vi "FEA_Model_Bounded_Regression.vi"(8 "error in (no error)":errorcluster, 11 "FEA_Model in":refnum<class "FEA_Model.lvclass">) -> (0 "error out":errorcluster, 3 "FEA_Model out":refnum<class "FEA_Model.lvclass">)   [LabVIEW 2021, in "FEA_Model.lvclass"]
uses:
  FEA_Model.lvclass
  FEA_Model.lvclass/FEA_Model.ctl
  <vilib>/Analysis/baseanly.llb/Real A x B.vi
  <vilib>/Analysis/baseanly.llb/Real Inverse Matrix.vi
  <vilib>/Analysis/NI_AALBase.lvlib
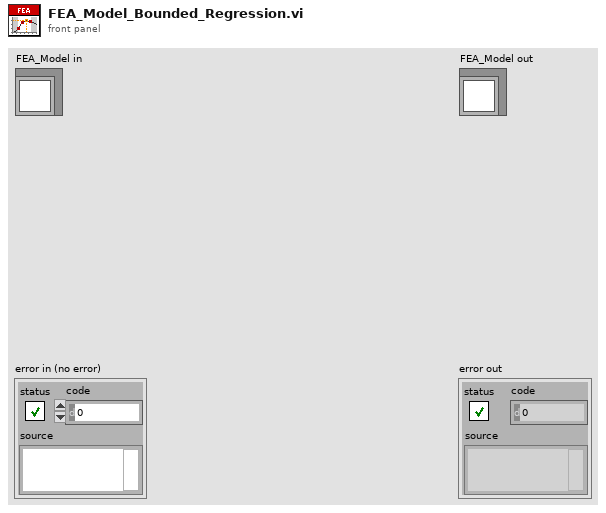
[diagram p1: front panel]
types:
  T1 = enum16{"Scalar Particle to Meter", "Scalar Node to Meter", "Scalar Meter to Particle", "Scalar Meter to Node", "Array Particle to Meter", "Array Node to Meter", "Array Meter to Particle", "Array Meter to Node"}
  T2 = typedef "NI_Matrix.lvlib/RealMatrix.ctl" = dbl[][]
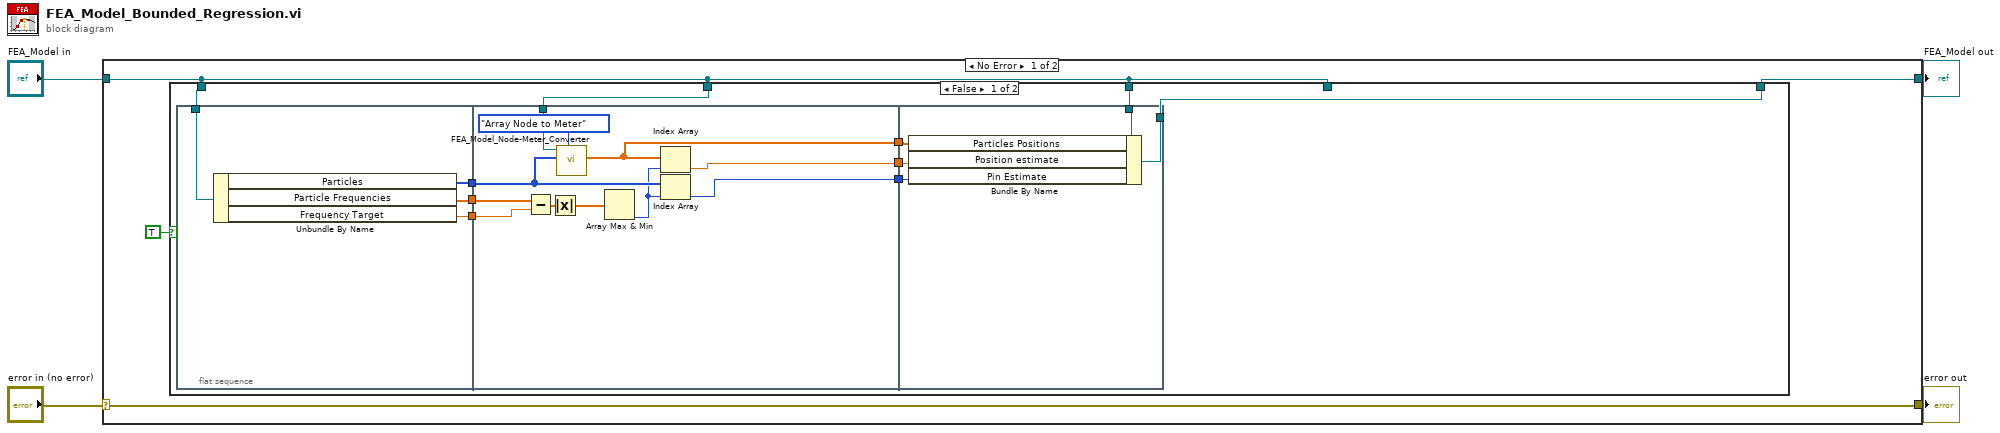
[diagram p0: block diagram]
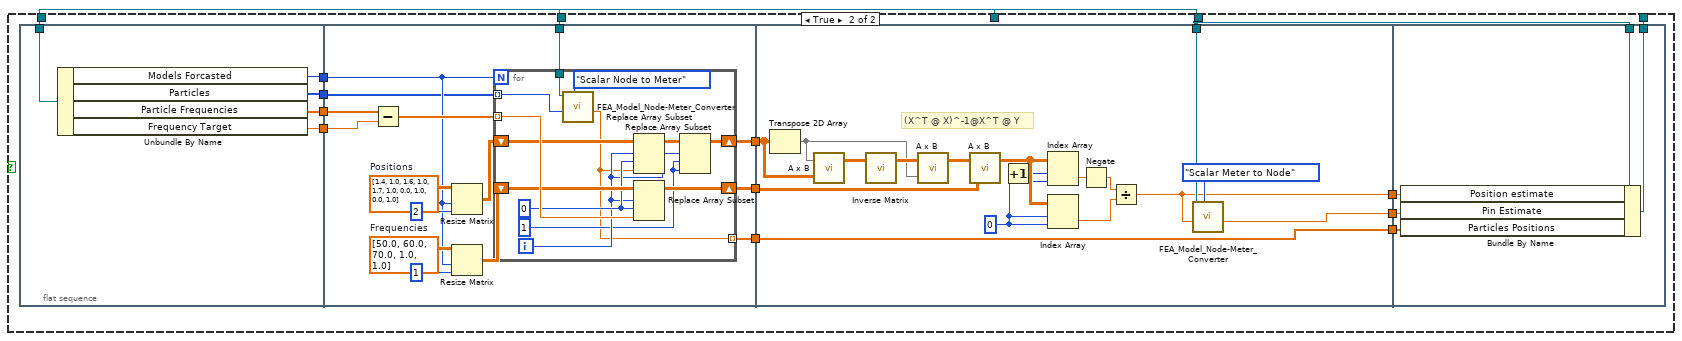
[diagram p2: hidden frame]
diagram:
  n1 = case shown="No Error" "error in (no error)" {
    selector: "error in (no error)" -> [w8 w107]
    tunnel: [w8 w107] -> w3
    tunnel: [w7 w106] -> w1
    tunnel: "FEA_Model in" -> [w6 w106]
    frame No Error {
      n2 = case shown="False" TRUE {
        tunnel: w6 -> [w15 w40]
        tunnel: [w12 w39] -> w7
        tunnel: w6 -> [_ _]
        tunnel: w6 -> [w14 _]
        tunnel: w6 -> [w13 _]
        frame False {
          n3 = flat-sequence {
            tunnel: [w19] -> w18
            tunnel: [w20] -> w17
            tunnel: [w21] -> w16
            tunnel: w13 -> [w22]
            tunnel: w14 -> [w27]
            tunnel: w18 -> [w33]
            tunnel: w17 -> [w32]
            tunnel: w16 -> [w28]
            tunnel: [w29] -> w11
            tunnel: [w25] -> w10
            tunnel: [w24] -> w9
            tunnel: w15 -> [w38]
            tunnel: [w37] -> w12
            tunnel: w11 -> [w36]
            tunnel: w10 -> [w35]
            tunnel: w9 -> [w34]
            frame #0 {
              n4 = Unbundle By Name(w22) -> ("Particles"=w21:i32[], "Particle Frequencies"=w20:dbl[], "Frequency Target"=w19:dbl)
            }
            frame #1 {
              n5 = Subtract(x=w32, y=w33) -> (x-y=w31:dbl[])
              n6 = Absolute Value(x=w31) -> (abs(x)=w30:dbl[])
              n7 = call "FEA_Model_Node-Meter_Converter.vi"("Conversion Mode"=T1."Array Node to Meter", "Array in"=w28, "FEA_Model in"=w27) -> ("Array out"=w24:dbl[])  [unwired: 5 in, 3 out]
              n8 = Array Max & Min(array=w30) -> (min index (indices)=w26:i32)  [unwired: 3 out]
              n9 = Index Array(array=w24, index=w26) -> (element=w25:dbl)
              n10 = Index Array(array=w28, index=w26) -> (element=w29:i32)
            }
            frame #2 {
              n11 = Bundle By Name(cluster=w38, "Particles Positions"=w34, "Position estimate"=w35, "Pin Estimate"=w36) -> (w37:refnum<class "FEA_Model.lvclass">)
            }
          }
        }
        frame True {
          n12 = flat-sequence {
            tunnel: [w51] -> w50
            tunnel: [w52] -> w49
            tunnel: [w53] -> w48
            tunnel: [w54] -> w47
            tunnel: w40 -> [w55]
            tunnel: [w70] -> w46
            tunnel: [w69] -> w45
            tunnel: w40 -> [w58]
            tunnel: w50 -> [w67]
            tunnel: w49 -> [w66]
            tunnel: w48 -> [w57]
            tunnel: w47 -> [w59]
            tunnel: [w56] -> w44
            tunnel: w46 -> [w100]
            tunnel: w45 -> [w95]
            tunnel: w40 -> [w88]
            tunnel: [w84] -> w43
            tunnel: [w85] -> w42
            tunnel: w44 -> [w87]
            tunnel: [w87] -> w41
            tunnel: w43 -> [w104]
            tunnel: w42 -> [w103]
            tunnel: w40 -> [w105]
            tunnel: [w102] -> w39
            tunnel: w41 -> [w101]
            frame #0 {
              n13 = Unbundle By Name(w55) -> ("Models Forcasted"=w54:i32, "Particles"=w53:i32[], "Particle Frequencies"=w52:dbl[], "Frequency Target"=w51:dbl)
            }
            frame #1 {
              w63 = dbl[][] [[50.0], [60.0], [70.0], [1.0], [1.0]]  # Frequencies
              w65 = dbl[][] [[1.4, 1.0], [1.6, 1.0], [1.7, 1.0], [0.0, 1.0], [0.0, 1.0]]  # Positions
              n14 = Subtract(x=w66, y=w67) -> (x-y=w68:dbl[])
              n15 = Resize Matrix(1:2 ("number of columns"), 2:w59, 4:w65) -> (0:w64:dbl[][])
              n16 = Resize Matrix(1:1, 2:w59, 4:w63) -> (0:w62:dbl[][])
              n17 = for {
                N: w59 -> [_]
                tunnel: w57 -> [w72] mode=indexing
                tunnel: w68 -> [w83] mode=indexing
                shift-right: [w79] -> w69
                shift-left: w62 -> [w81]
                shift-right: [w77] -> w70
                shift-left: w64 -> [w82]
                tunnel: w58 -> [w74]
                tunnel: [w73] -> w56 mode=indexing
                i -> [w76]
                w75 = 1 ("disabled index (row)")
                w80 = 0 ("disabled index (col)")
                n18 = call "FEA_Model_Node-Meter_Converter.vi"("Conversion Mode"=T1."Scalar Node to Meter", "Scalar in"=w72, "FEA_Model in"=w74) -> ("Scalar out"=w73:dbl)  [unwired: 5 in, 3 out]
                n19 = Replace Array Subset(array=w82, new element=w73, index (row)=w76, index (col)=w80) -> (w78:dbl[][])
                n20 = Replace Array Subset(array=w81, new element=w83, index (row)=w76, index (col)=w80) -> (w79:dbl[][])
                n21 = Replace Array Subset(array=w78, new element=w75, index (row)=w76, index (col)=w75) -> (w77:dbl[][])
              }
            }
            frame #2 {
              w91 = 0 ("index (row)")
              # "(X^T @ X)^-1@X^T @ Y"
              n22 = Transpose 2D Array(2D array=w100) -> (transposed array=w97:dbl[][])
              n23 = call-poly <vilib>:"A x B.vi"("B"=w100, "A"=w97) -> ("A x B"=w99:T2)  [unwired: 1 out]
              n24 = call-poly <vilib>:"Inverse Matrix.vi"("Input Matrix"=w99) -> ("Inverse Matrix"=w98:T2)  [unwired: 1 in, 1 out]
              n25 = call-poly <vilib>:"A x B.vi"("B"=w97, "A"=w98) -> ("A x B"=w96:T2)  [unwired: 1 out]
              n26 = call-poly <vilib>:"A x B.vi"("B"=w95, "A"=w96) -> ("A x B"=w94:T2)  [unwired: 1 out]
              n27 = Increment(x=w91) -> (x+1=w92:i32)
              n28 = Index Array(array=w94, index (row)=w92, index (col)=w91) -> (element=w90:dbl)
              n29 = Index Array(array=w94, index (row)=w91, index (col)=w91) -> (element=w93:dbl)
              n30 = Negate(x=w90) -> (-x=w89:dbl)
              n31 = Divide(x=w89, y=w93) -> (x/y=w84:dbl)
              n32 = call "FEA_Model_Node-Meter_Converter.vi"("Conversion Mode"=T1."Scalar Meter to Node", "Scalar in"=w84, "FEA_Model in"=w88) -> ("Scalar out"=w85:dbl)  [unwired: 5 in, 3 out]
            }
            frame #3 {
              n33 = Bundle By Name(cluster=w105, "Position estimate"=w104, "Pin Estimate"=w103, "Particles Positions"=w101) -> (w102:refnum<class "FEA_Model.lvclass">)
            }
          }
        }
      }
    }
    frame Error {
    }
  }
  "error out" <- w3
  "FEA_Model out" <- w1
